vi "SetBitsInByte (SubVI).vi"(1 "Iput Byte":u8=54 format="%08b", 2 "Bitsmask":u8=6 format="%08b", 3 "Bits to set":u8=4 format="%08b") -> (0 "Output Byte":u8=54 format="%08b")   [LabVIEW 2017]
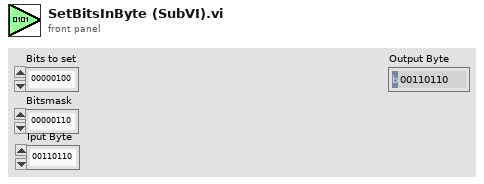
[diagram p1: front panel]
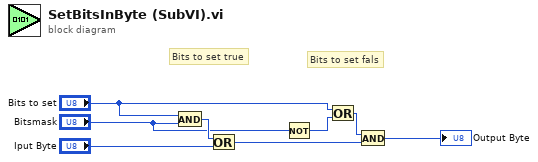
[diagram p0: block diagram]
diagram:
  # "Bits to set fals"
  # "Bits to set true"
  n1 = And(x="Bits to set", y="Bitsmask") -> (x .and. y?=w8:u8)
  n2 = Or(x=w8, y="Iput Byte") -> (x .or. y?=w2:u8)
  n3 = Not(x="Bitsmask") -> (.not. x?=w6:u8)
  n4 = Or(x="Bits to set", y=w6) -> (x .or. y?=w3:u8)
  n5 = And(x=w3, y=w2) -> (x .and. y?=→"Output Byte":u8)
